vi "niRFSysCalReader Fetch Receiver Offset.vi"(8 "error in":errorcluster, 9 "Reference Level (dBm)":dbl, 10 "Frequency (Hz)":dbl, 11 "niRFSysCalReader Handle":T1) -> (0 "error out":errorcluster, 2 "Receiver Offset (dB)":dbl, 3 "niRFSysCalReader Handle out":T1)   [LabVIEW 2016, in "niRFSysCalReader.lvlib"]
doc: "Returns the receiver offset for the specified frequency and reference level. \n\n<b>Note:</b> To accurately measure the power at the receiver's input port, make the signal analyzer reference level attribute equal to the input <b>Reference Level (dBm)</b>'s value and make the signal analyzer's external gain attribute or signal analyzer's reference level offset attribute equal to the result of negating the returned <b>Receiver Offset (dB)</b> value.\ni.e.\nSignal Analyzer's Reference Level = Reference Level\nSignal Analyzer's External Gain = -1 * Receiver Offset"
uses:
  niRFSysCalReader.lvlib
  INCLUDES/niRFSysCalReader Handle.ctl
  INCLUDES/niRFSysCalReader Core States.ctl
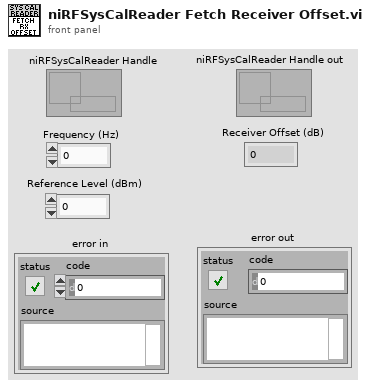
[diagram p1: front panel]
types:
  T1 = typedef "niRFSysCalReader.lvlib/niRFSysCalReader Handle.ctl" = refnum<data-value>
  T2 = typedef "niRFSysCalReader.lvlib/niRFSysCalReader Core States.ctl" = enum16{"Initialize", "Interpolator State", "Add CalData", "Get CalData", "Remove Pathloss", "Close"}
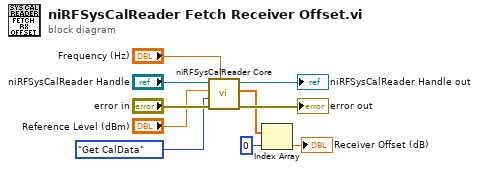
[diagram p0: block diagram]
diagram:
  n1 = call "niRFSysCalReader Core.vi"("Frequency (Hz)"="Frequency (Hz)", "error in"="error in", "niRFSysCalReader State"=niRFSysCalReader_Core_States."Get CalData" ("Cal Storage"), "Power (dBm)"="Reference Level (dBm)", "niRFSysCalReader Handle"="niRFSysCalReader Handle") -> ("error out"=→"error out":errorcluster, "CalData Out"=w3:dbl[], "niRFSysCalReader Handle out"=→"niRFSysCalReader Handle out":T1)  [unwired: 4 in]
  n2 = Index Array(array=w3, index=0) -> (element=→"Receiver Offset (dB)":dbl)
